vi "bindata to image.vi"(8 "error in (no error)":errorcluster, 9 "name":string="img", 10 "binary data in":u8[](array[numeric]), 11 "JSON in":string) -> (0 "error out":errorcluster, 2 "img_type":string, 3 "img out":T1)   [LabVIEW 2018, in "LV-0mq-Julia_roundtrip-lib.lvlib"]
uses:
  LV-0mq-Julia_roundtrip-lib.lvlib
  <vilib>/picture/picture.llb/imagedata.ctl
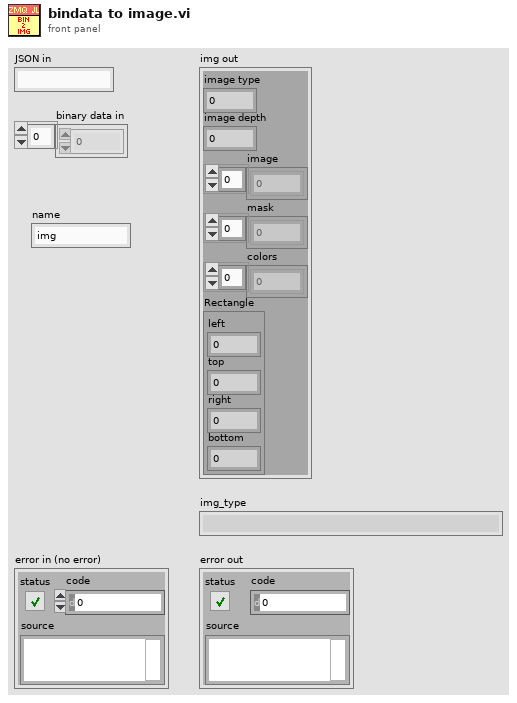
[diagram p1: front panel]
types:
  T1 = typedef "imagedata.ctl" = cluster{"image type":i32, "image depth":i32, "image":u8[], "mask":u8[], "colors":u32[], "Rectangle":cluster{"left":i16, "top":i16, "right":i16, "bottom":i16}}
  T2 = typedef "LV-0mq-Julia_roundtrip-lib.lvlib/Bindata&description.ctl" = cluster{"bindata_descr":T3[], "bindata":u8[]}
  T3 = typedef "LV-0mq-Julia_roundtrip-lib.lvlib/Bindata description.ctl" = cluster{"nofbytes":i32, "numtype":string, "start":i32, "arrdims":i32[], "kwarg_name":string, "category":string}
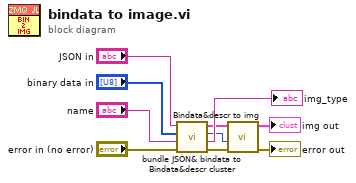
[diagram p0: block diagram]
diagram:
  n1 = call "bundle JSON& bindata to Bindata&descr cluster.vi"("error in (no error)"="error in (no error)", "name"="name", "binary data received"="binary data in", "JSON received"="JSON in") -> ("error out"=w2:errorcluster, "img_type"=→"img_type":string, "index"=w4:i32, "Bindata & descr out"=w3:T2)  [unwired: 4 in]
  n2 = call "Bindata&descr to img.vi"("error in (no error)"=w2, "bindata_descr index"=w4, "Bindata & descr in"=w3) -> ("error out"=→"error out":errorcluster, "img out"=→"img out":T1)  [unwired: 7 in]
